vi "EIP INIT.vi"(0 "Subband":i32=3, 1 "Center Freq (GHz)":dbl=140.2 format="%.3f") -> ()   [LabVIEW 2009]
doc: "This VI initializes the EIP fregquncy counter. The only input variable is the central frequncy boolean. If true the scan cnetralfrequency is set to 140GhZ. THis is the defualt"
uses:
  MWC Global.vi
panel:
  out "Returned Setup String":string
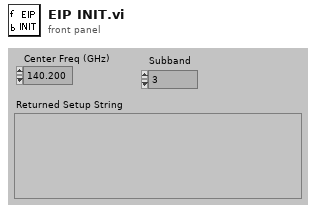
[diagram p1: front panel]
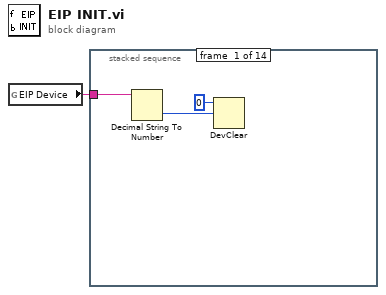
[diagram p0: block diagram]
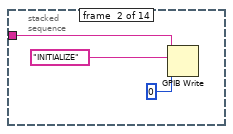
[diagram p2: hidden frame]
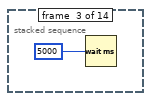
[diagram p3: hidden frame]
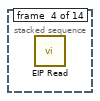
[diagram p4: hidden frame]
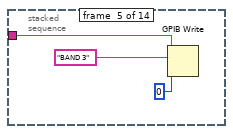
[diagram p5: hidden frame]
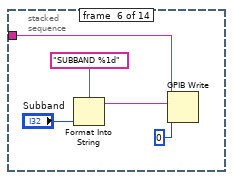
[diagram p6: hidden frame]
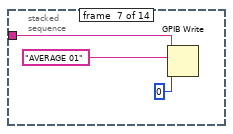
[diagram p7: hidden frame]
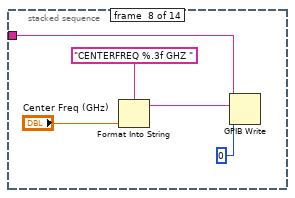
[diagram p8: hidden frame]
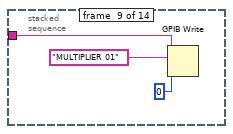
[diagram p9: hidden frame]
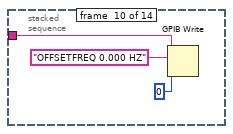
[diagram p10: hidden frame]
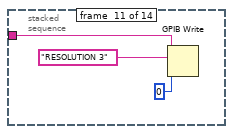
[diagram p11: hidden frame]
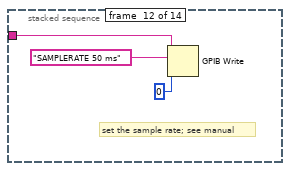
[diagram p12: hidden frame]
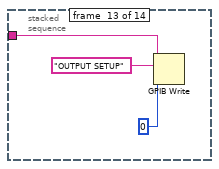
[diagram p13: hidden frame]
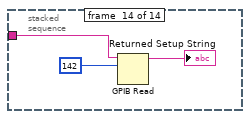
[diagram p14: hidden frame]
diagram:
  n1 = global read "MWC Global.vi" "EIP Device"() -> (w1:string)
  n2 = stacked-sequence {
    tunnel: w1 -> [w4 w6 _ _ w10 w16 w18 w24 w26 w29 w32 w35 w38 w40]
    frame #0 {
      n3 = Decimal String To Number(string=w4) -> (number=w3:i32)  [unwired: 2 in, 1 out]
      n4 = DevClear(3:w3, 4:0 ("bus")) -> ()  [unwired: 1 in, 2 out]
    }
    frame #1 {
      n5 = GPIB Write(0:w6, 1:"INITIALIZE", 2:0) -> ()  [unwired: 2 in, 2 out]
    }
    frame #2 {
      n6 = Wait (ms)(milliseconds to wait=u32 5000) -> ()  [unwired: 1 out]
    }
    frame #3 {
      n7 = call "EIP Read.vi"() -> ()  [unwired: 1 out]
    }
    frame #4 {
      n8 = GPIB Write(0:w10, 1:"BAND 3", 2:0) -> ()  [unwired: 2 in, 2 out]
    }
    frame #5 {
      n9 = Format Into String(format string="SUBBAND %1d", "Subband") -> (resulting string=w13:string)  [unwired: 2 in, 1 out]
      n10 = GPIB Write(0:w16, 1:w13, 2:0) -> ()  [unwired: 2 in, 2 out]
    }
    frame #6 {
      n11 = GPIB Write(0:w18, 1:"AVERAGE 01", 2:0) -> ()  [unwired: 2 in, 2 out]
    }
    frame #7 {
      n12 = Format Into String(format string="CENTERFREQ %.3f GHZ ", "Center Freq (GHz)") -> (resulting string=w20:string)  [unwired: 2 in, 1 out]
      n13 = GPIB Write(0:w24, 1:w20, 2:0) -> ()  [unwired: 2 in, 2 out]
    }
    frame #8 {
      n14 = GPIB Write(0:w26, 1:"MULTIPLIER 01", 2:0) -> ()  [unwired: 2 in, 2 out]
    }
    frame #9 {
      n15 = GPIB Write(0:w29, 1:"OFFSETFREQ 0.000 HZ", 2:0) -> ()  [unwired: 2 in, 2 out]
    }
    frame #10 {
      n16 = GPIB Write(0:w32, 1:"RESOLUTION 3", 2:0) -> ()  [unwired: 2 in, 2 out]
    }
    frame #11 {
      # "set the sample rate; see manual"
      n17 = GPIB Write(0:w35, 1:"SAMPLERATE 50 ms", 2:0) -> ()  [unwired: 2 in, 2 out]
    }
    frame #12 {
      n18 = GPIB Write(0:w38, 1:"OUTPUT SETUP", 2:0) -> ()  [unwired: 2 in, 2 out]
    }
    frame #13 {
      n19 = GPIB Read(0:w40, 1:142) -> (5:→"Returned Setup String":string)  [unwired: 3 in, 2 out]
    }
  }
